vi "Stop EHL (library variable).vi"() -> ()   [LabVIEW 2023, in "Error Manager.lvlib" / "New Error Window.lvlib"]
uses:
  New Error Window.lvlib
panel:
  out "Stop EHL?":bool
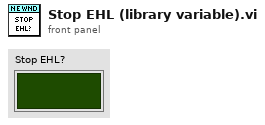
[diagram p1: front panel]
diagram:
